vi "PH Radial Imagehash.vi"(11 "Image Path":path=path "C:/Users/Matthew/Clients/Users Group/Coding Challenge/Submissions/drt.bmp") -> (3 "Digest":cluster{"*id":u32, "*Coeffs":u32, "size":i32})   [LabVIEW 2020, in "Perceptual Hash Comparison.lvclass"]
uses:
  Perceptual Hash Comparison.lvclass
  phash DLL/pHash.dll
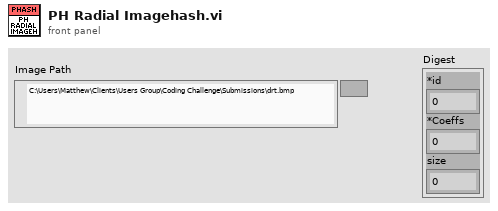
[diagram p1: front panel]
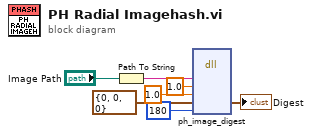
[diagram p0: block diagram]
diagram:
  n1 = Path To String(path="Image Path") -> (string=w6:string)
  n2 = dll-call lib="D:/code/labview/labview-reddit-coding-challenge-june-2021/Perceptual Hash Comparison/phash DLL/pHash.dll" fn="ph_image_digest"("file"=w6, "sigma"=1.0, "gamma"=1.0, "digest"=cluster{"*id":u32, "*Coeffs":u32, "size":i32} {"*id"=0, "*Coeffs"=0, "size"=0} ("Digest In"), "N"=180) -> ("digest"=→"Digest":cluster{"*id":u32, "*Coeffs":u32, "size":i32})  [unwired: 8 in, 2 out]
